vi "Schrittmotor_Nema17.vi"(1 "Schrittweite  eingeben":dbl=18.0 format="%#_13g", 8 "x_Ellipse":u8=40 max=200 step=1, 10 "RN-Motor - RS232 2":refnum<visa-resource-name>="COM5", 11 "Motor an?":bool=TRUE) -> (3 "Schrittweite rechnen":dbl=18.0 format="%#_13g")   [LabVIEW 2014]
uses:
  <vilib>/Instr/_visa.llb/VISA Configure Serial Port (Instr).vi
  <vilib>/DAQmx/write.llb/DAQmx Write (Digital Bool 1Line 1Point).vi
panel:
  out "error out 7":errorcluster
  out "error out 6":errorcluster
  in  "Schrittgeschwindigkeit":u8=20
  in  "Stromstärke in mA / 10":u8=40 max=200 step=1
  in  "Motorwahl":string(combo)="0"
  # "x>= 100, nach links\nx<100, nach rechts"
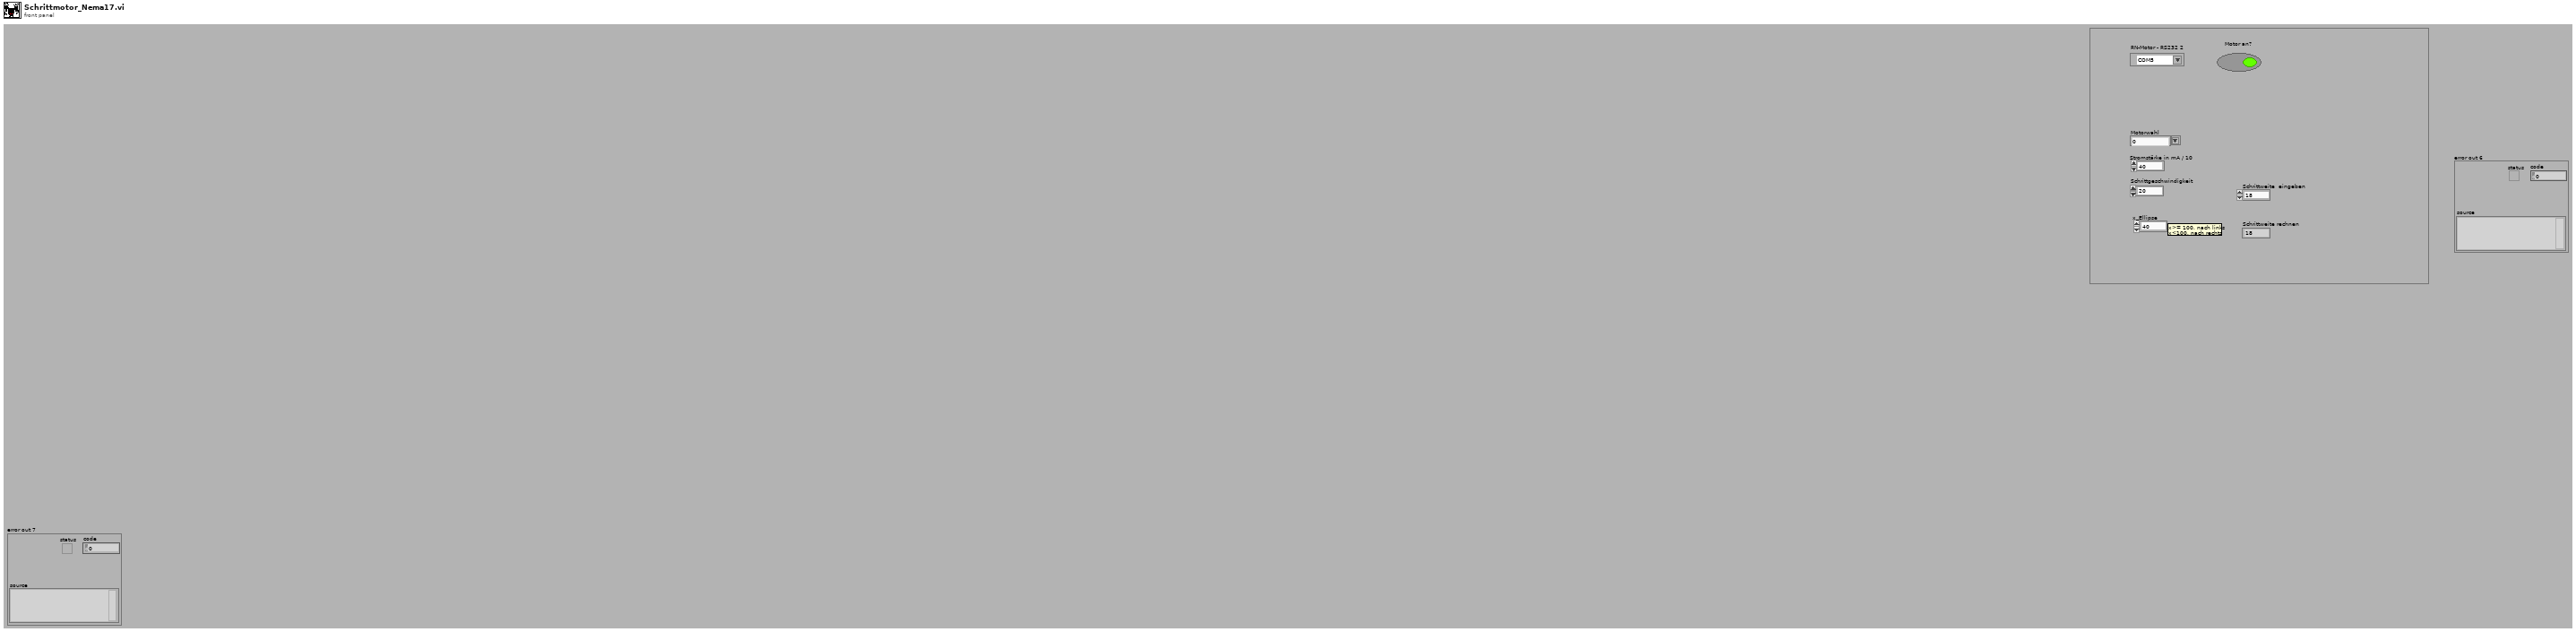
[diagram p1: front panel]
types:
  T1 = cluster{"VISA resource name out":refnum<visa-resource-name>, "Motorwahl":string, "Schrittweite (°)":dbl, "error out":errorcluster}
  T2 = cluster{"VISA resource name out":refnum<visa-resource-name>, "Gesendeter Code":string, "Schrittweite  eingeben  ":dbl, "error out":errorcluster}
  T3 = cluster{"VISA resource name out":refnum<visa-resource-name>, "Gesendeter Code":string, "error out":errorcluster}
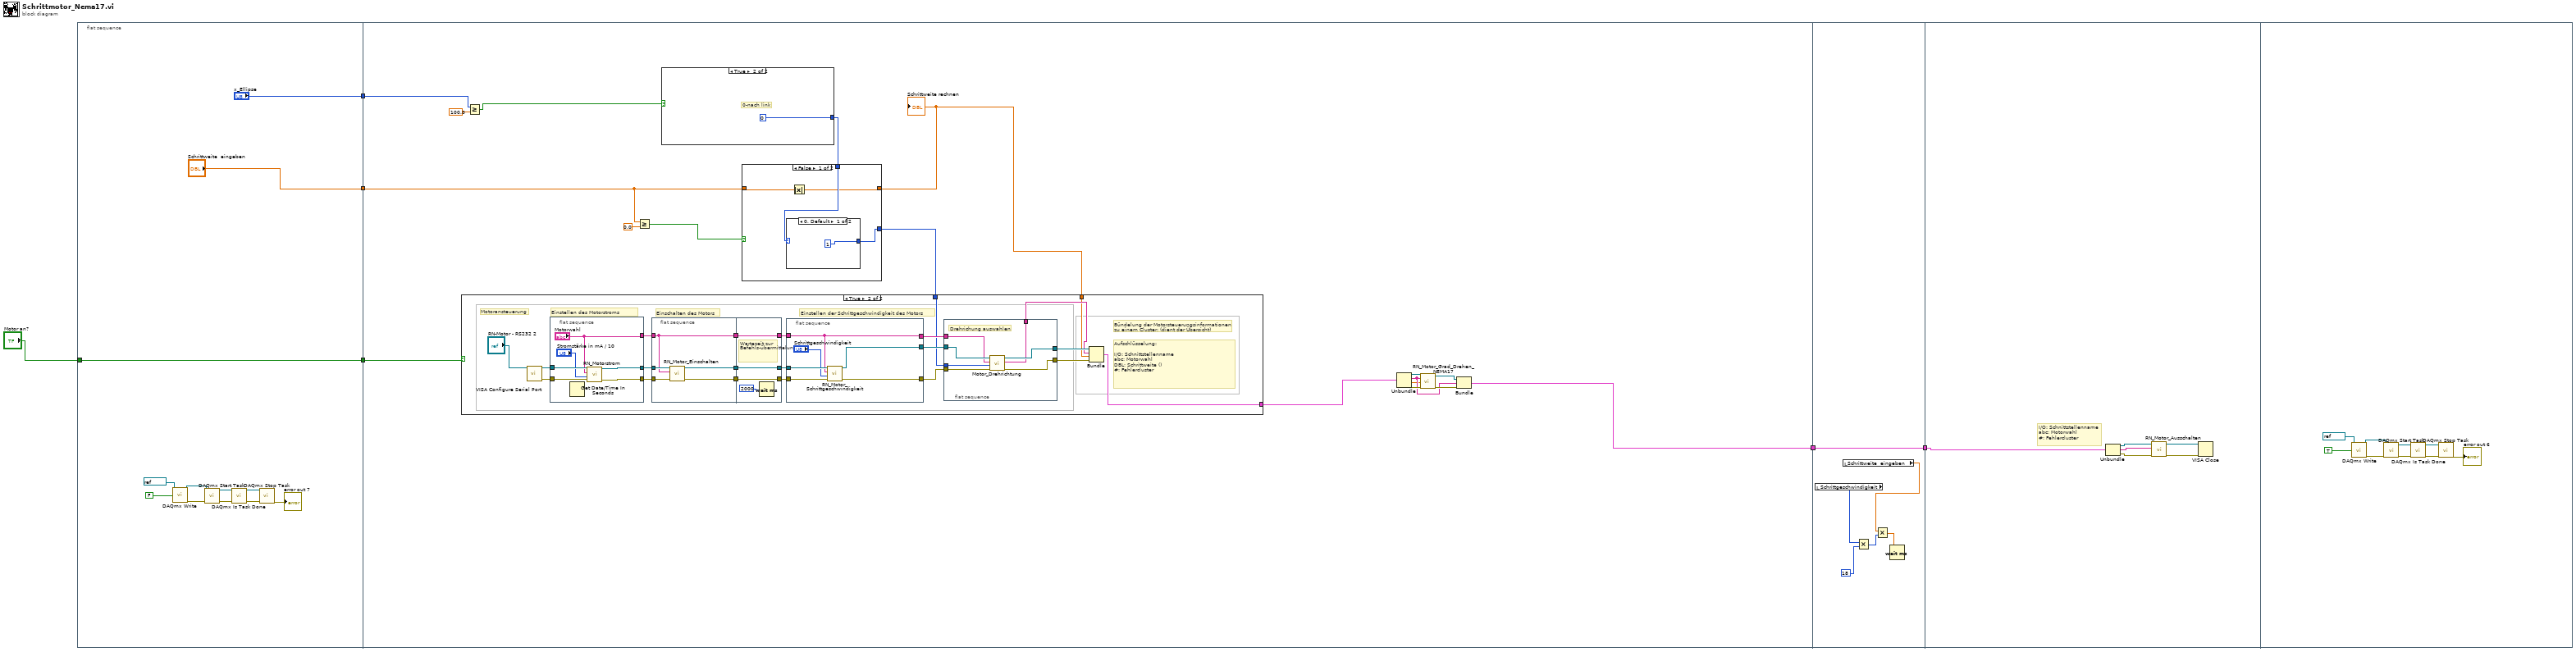
[diagram p0: block diagram]
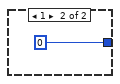
[diagram p2: hidden frame]
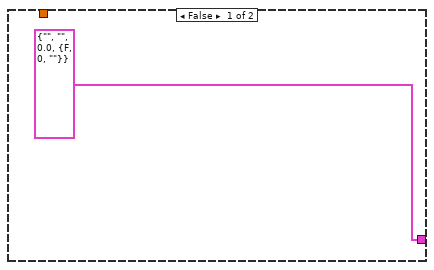
[diagram p4: hidden frame]
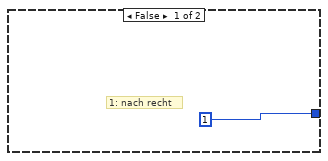
[diagram p5: hidden frame]
diagram:
  n1 = flat-sequence {
    tunnel: "Motor an?" -> [w18]
    tunnel: [w18] -> w5
    tunnel: ["Schrittweite  eingeben"] -> w2
    tunnel: ["x_Ellipse"] -> w1
    tunnel: [w36] -> w4
    tunnel: w5 -> [w35]
    tunnel: w2 -> [w23]
    tunnel: w1 -> [w21]
    tunnel: w4 -> [w102]
    tunnel: [w102] -> w3
    tunnel: w3 -> [w108]
    frame #0 {
      n2 = call-poly <vilib>:"DAQmx Write.vi"("task/channels in"=refnum<k21> "LED", "data"=FALSE) -> ("task out"=w17:refnum<k21>, "error out"=w16:errorcluster)  [unwired: 11 in, 1 out]
      n3 = call <vilib>:"DAQmx Start Task.vi"("task/channels in"=w17, "error in"=w16) -> ("task out"=w15:refnum<k21>, "error out"=w14:errorcluster)  [unwired: 12 in]
      n4 = call <vilib>:"DAQmx Is Task Done.vi"("task/channels in"=w15, "error in"=w14) -> ("task out"=w13:refnum<k21>, "error out"=w12:errorcluster)  [unwired: 11 in, 1 out]
      n5 = call <vilib>:"DAQmx Stop Task.vi"("task/channels in"=w13, "error in"=w12) -> ("error out"=→"error out 7":errorcluster)  [unwired: 12 in, 1 out]
    }
    frame #1 {
      n6 = Greater Or Equal?(x=w21, y=100.0) -> (x >= y?=w19:bool)
      n7 = Greater Or Equal?(x=w23, y=0.0) -> (x >= y?=w26:bool)
      n8 = case shown="True" w19 {
        tunnel: [u8 1 ("Drehrichtung") 0] -> w25
        frame False {
          # "1: nach recht"
        }
        frame True {
          # "0-nach link"
        }
      }
      n9 = case shown="False" w26 {
        tunnel: w25 -> [w40 w44]
        tunnel: [w39 w44] -> w24
        tunnel: [w37 w43] -> w22
        tunnel: w23 -> [w38 w43]
        frame False {
          n10 = case shown="0, Default" w40 {
            tunnel: [1 0] -> w39
            frame 0, Default {
            }
            frame 1 {
            }
          }
          n11 = Absolute Value(x=w38) -> (abs(x)=w37:dbl)
        }
        frame True {
        }
      }
      "Schrittweite rechnen" <- w22
      n12 = case shown="True" w35 {
        tunnel: [T1 {"VISA resource name out"="", "Motorwahl"="", "Schrittweite (°)"=0.0, "error out"={"status"=FALSE, "code"=0, "source"=""}} ("output cluster") w48] -> w34
        tunnel: w22 -> [_ w47]
        tunnel: w24 -> [_ w46]
        frame False {
        }
        frame True {
          # "Aufschlüsselung:\n\nI/O: Schnittstellenname\nabc: Motorwahl \nDBL: Schrittweite ()\n#: Fehlercluster"
          # "Bündelung der Motorsteuerungsinformationen \nzu einem Cluster: (dient der Übersicht)"
          # "Einstellen der Schrittgeschwindigkeit des Motors"
          # "Einschalten des Motors"
          # "Einstellen des Motorstroms"
          # "Motoransteuerung"
          n13 = call-poly "VISA Configure Serial Port"("VISA resource name"="RN-Motor - RS232 2") -> ("VISA resource name out"=w63:refnum<visa-resource-name>, "error out"=w62:errorcluster)  [unwired: 13 in]
          n14 = flat-sequence {
            tunnel: w63 -> [w94]
            tunnel: w62 -> [w93]
            tunnel: [w91] -> w61
            tunnel: [w90] -> w60
            tunnel: ["Motorwahl"] -> w56
            frame #0 {
              n15 = Get Date/Time In Seconds() -> ()  [unwired: 1 out]
              n16 = call "RN_Motorstrom.vi"("error in"=w93, "Stromstärke in mA / 10"="Stromstärke in mA / 10", "Motorwahl"="Motorwahl", "VISA resource name in"=w94) -> ("error out"=w90:errorcluster, "VISA resource name out"=w91:refnum<visa-resource-name>)  [unwired: 3 in, 1 out]
            }
          }
          n17 = flat-sequence {
            tunnel: w61 -> [w84]
            tunnel: w60 -> [w83]
            tunnel: w56 -> [w80]
            tunnel: [w82] -> w66
            tunnel: [w81] -> w65
            tunnel: [w80] -> w64
            tunnel: [w87] -> w58
            tunnel: [w88] -> w59
            tunnel: w66 -> [w88]
            tunnel: w65 -> [w87]
            tunnel: [w85] -> w57
            tunnel: w64 -> [w85]
            frame #0 {
              n18 = call "RN_Motor_Einschalten.vi"("error in"=w83, "Motorwahl"=w80, "VISA resource name in"=w84) -> ("error out"=w81:errorcluster, "VISA resource name out"=w82:refnum<visa-resource-name>)  [unwired: 3 in, 2 out]
            }
            frame #1 {
              # "Wartezeit zur Befehls-übermittelung"
              n19 = Wait (ms)(milliseconds to wait=u32 2000) -> ()  [unwired: 1 out]
            }
          }
          n20 = flat-sequence {
            tunnel: w59 -> [w79]
            tunnel: w58 -> [w78]
            tunnel: [w76] -> w52
            tunnel: [w75] -> w54
            tunnel: w57 -> [w74]
            tunnel: [w74] -> w53
            frame #0 {
              n21 = call "RN_Motor_Schrittgeschwindigkeit.vi"("error in"=w78, "Schrittgeschwindigkeit"="Schrittgeschwindigkeit", "Motorwahl"=w74, "VISA resource name in"=w79) -> ("error out"=w76:errorcluster, "VISA resource name out"=w75:refnum<visa-resource-name>)  [unwired: 3 in, 1 out]
            }
          }
          n22 = flat-sequence {
            tunnel: [w73] -> w55
            tunnel: w54 -> [w72]
            tunnel: w53 -> [w71]
            tunnel: w52 -> [w70]
            tunnel: [w69] -> w51
            tunnel: [w68] -> w49
            tunnel: w46 -> [w67]
            frame #0 {
              # "Drehrichung auswahlen"
              n23 = call "Motor_Drehrichtung.vi"("error in"=w70, "drehrichtung"=w67, "Motorwahl"=w71, "VISA resource name in"=w72) -> ("error out"=w69:errorcluster, "Gesendeter Code"=w68:string, "VISA resource name out"=w73:refnum<visa-resource-name>)  [unwired: 5 in]
            }
          }
          n24 = Bundle("VISA resource name out"=w55, "Gesendeter Code"=w49, "Schrittweite  eingeben"=w47, "error out"=w51) -> (w48:T2)  [unwired: 1 in]
        }
      }
      n25 = Unbundle(w34) -> ("VISA resource name out"=w33:refnum<visa-resource-name>, "Gesendeter Code"=w29:string, "Schrittweite  eingeben"=w28:dbl, "error out"=w32:errorcluster)
      n26 = call "RN_Motor_Grad_Drehen_NEMA17.vi"("error in"=w32, "Drehwinkel (°)"=w28, "Motorwahl"=w29, "VISA resource name in"=w33) -> ("error out"=w30:errorcluster, "VISA resource name out"=w31:refnum<visa-resource-name>)  [unwired: 3 in, 1 out]
      n27 = Bundle("VISA resource name out"=w31, "Gesendeter Code"=w29, "error out"=w30) -> (w36:T3)  [unwired: 1 in]
    }
    frame #2 {
      n28 = local read "Schrittgeschwindigkeit"() -> (w100:u8)
      n29 = local read "Schrittweite  eingeben"() -> (w97:dbl)
      n30 = Multiply(x=w100, y=u32 18 ("milliseconds to wait")) -> (x*y=w99:u32)
      n31 = Multiply(x=w97, y=w99) -> (x*y=w98:dbl)
      n32 = Wait (ms)(milliseconds to wait=w98) -> ()  [unwired: 1 out]
    }
    frame #3 {
      # "I/O: Schnittstellenname\nabc: Motorwahl \n#: Fehlercluster"
      n33 = Unbundle(w108) -> ("VISA resource name out"=w104:refnum<visa-resource-name>, "Gesendeter Code"=w103:string, "error out"=w105:errorcluster)
      n34 = call "RN_Motor_Ausschalten.vi"("error in"=w105, "Motorwahl"=w103, "VISA resource name in"=w104) -> ("error out"=w106:errorcluster, "VISA resource name out"=w107:refnum<visa-resource-name>)  [unwired: 3 in, 2 out]
      n35 = VISA Close(VISA resource name=w107, error in (no error)=w106) -> ()  [unwired: 1 out]
    }
    frame #4 {
      n36 = call-poly <vilib>:"DAQmx Write.vi"("task/channels in"=refnum<k21> "LED", "data"=TRUE) -> ("task out"=w117:refnum<k21>, "error out"=w116:errorcluster)  [unwired: 11 in, 1 out]
      n37 = call <vilib>:"DAQmx Start Task.vi"("task/channels in"=w117, "error in"=w116) -> ("task out"=w115:refnum<k21>, "error out"=w114:errorcluster)  [unwired: 12 in]
      n38 = call <vilib>:"DAQmx Is Task Done.vi"("task/channels in"=w115, "error in"=w114) -> ("task out"=w113:refnum<k21>, "error out"=w112:errorcluster)  [unwired: 11 in, 1 out]
      n39 = call <vilib>:"DAQmx Stop Task.vi"("task/channels in"=w113, "error in"=w112) -> ("error out"=→"error out 6":errorcluster)  [unwired: 12 in, 1 out]
    }
  }
